vi "PWM Set Frequency.vi"(7 "pPrecision":u16[](array[numeric])=[0, 0, 0, 0, 0, 0, 0, 0], 9 "pPrescaler":u16[](array[numeric])=[0, 0, 0, 0, 0, 0, 0, 0], 10 "ChannelMask":u8, 11 "DevHandle":i32) -> (1 "pPrescaler out":u16[](array[numeric]), 3 "function return":i32, 5 "pPrecision out":u16[](array[numeric]))   [LabVIEW 2010, in "usb2pwm.lvlib"]
doc: "int WINAPI PWM_SetFrequency(int DevHandle,unsigned char ChannelMask,unsigned short *pPrescaler,unsigned short *pPrecision);"
uses:
  usb2pwm.lvlib
  USB2XXX/trunk/USB2XXX/USB2XXX/vs2019/Release/USB2XXX.dll
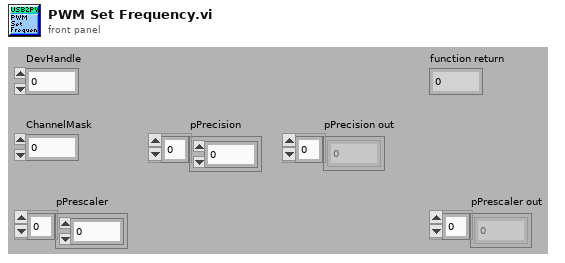
[diagram p1: front panel]
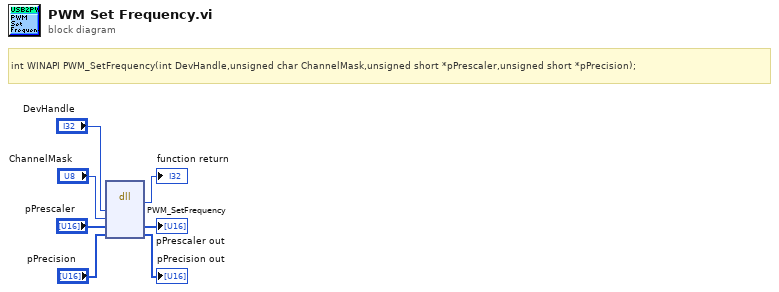
[diagram p0: block diagram]
diagram:
  # "int WINAPI PWM_SetFrequency(int DevHandle,unsigned char ChannelMask,unsigned short *pPrescaler,unsigned short *pPrecision);"
  n1 = dll-call lib="E:/Projects/USB2XXX/trunk/USB2XXX/USB2XXX/vs2019/Release/USB2XXX.*" fn="PWM_SetFrequency"("DevHandle"="DevHandle", "ChannelMask"="ChannelMask", "pPrescaler"="pPrescaler", "pPrecision"="pPrecision") -> (→"function return":i32, "pPrescaler"=→"pPrescaler out":u16[], "pPrecision"=→"pPrecision out":u16[])  [unwired: 5 in, 2 out]
